vi "Read.vi"(8 "error in (no error)":errorcluster, 11 "Keithley 2100 in":refnum<class "Keithley 2100.lvclass">) -> (0 "error out":errorcluster, 1 "Unit":string, 2 "Measure":dbl, 3 "Keithley 2100 out":refnum<class "Keithley 2100.lvclass">, 4 "Channel":i32)   [LabVIEW 2020, in "Keithley 2100.lvclass"]
uses:
  Keithley 2100.lvclass
  C:/Sandbox/Git_Sandbox/WiSpry Test Framework source code (LV20)/WiSpry Test Framework/Instruments/Instrument.lvclass
  C:/Sandbox/Git_Sandbox/WiSpry Test Framework source code (LV20)/WiSpry Test Framework/Instruments/Digital Multimeter/Digital Multimeter.lvclass
  Digital Multimeter.lvclass/Digital Multimeter.ctl
  Instrument.lvclass/Instrument.ctl
  Instrument.lvclass
  <instrlib>/Keithley 2100 Series/Keithley 2100 Series.lvlib
  Digital Multimeter.lvclass
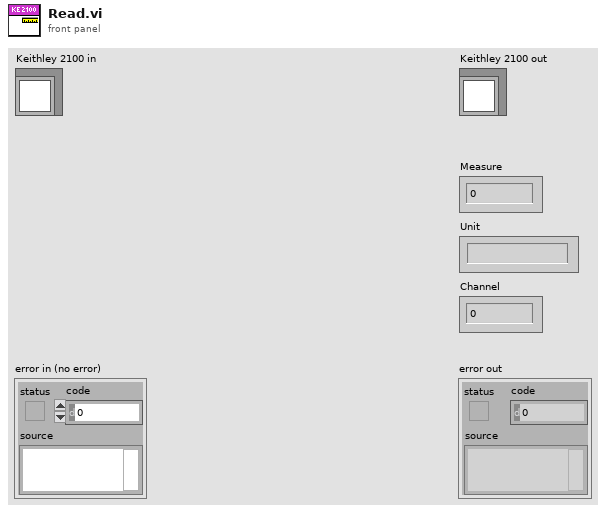
[diagram p1: front panel]
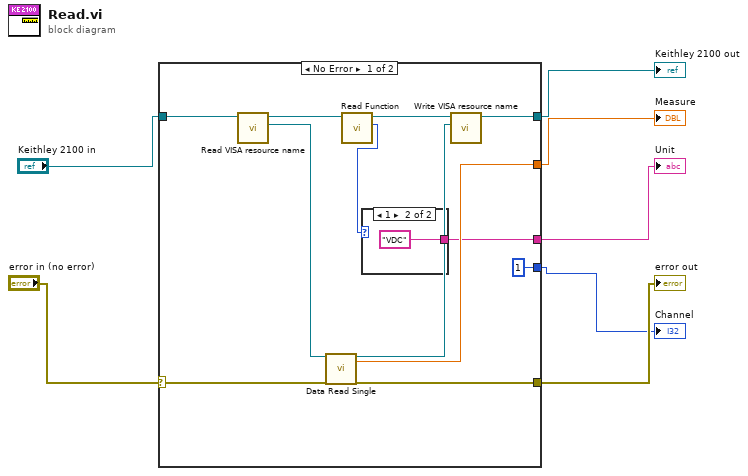
[diagram p0: block diagram]
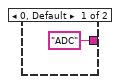
[diagram p2: hidden frame]
diagram:
  n1 = case shown="No Error" "error in (no error)" {
    selector: "error in (no error)" -> [w17 w23]
    tunnel: [w14 w23] -> w3
    tunnel: "Keithley 2100 in" -> [w19 w22]
    tunnel: [w18 w22] -> w4
    tunnel: [w13 _] -> w5
    tunnel: [1 ("Channel") _] -> w1
    tunnel: [w9 _] -> w2
    frame No Error {
      n2 = call "Read VISA resource name.vi"("Instrument in"=w19) -> ("VISA resource name"=w16:refnum<visa-resource-name>, "Instrument out"=w12:refnum<class "Keithley 2100.lvclass">)  [unwired: 9 in]
      n3 = call <instrlib>:"Data Read Single.vi"("VISA resource name"=w16, "error in (no error)"=w17) -> ("VISA resource name out"=w15:refnum<visa-resource-name>, "Measurement"=w13:dbl, "error out"=w14:errorcluster)  [unwired: 15 in]
      n4 = call "Read Function.vi"("Digtal Multimeter in"=w12) -> ("Function"=w10:u16, "Digtal Multimeter out"=w11:refnum<class "Keithley 2100.lvclass">)  [unwired: 9 in]
      n5 = case shown="1" w10 {
        tunnel: ["ADC" ("Unit") "VDC" ("Unit")] -> w9
        frame 0, Default {
        }
        frame 1 {
        }
      }
      n6 = call "Write VISA resource name.vi"("VISA resource name"=w15, "Instrument in"=w11) -> ("Instrument out"=w18:refnum<class "Keithley 2100.lvclass">)  [unwired: 9 in]
    }
    frame Error {
    }
  }
  "error out" <- w3
  "Keithley 2100 out" <- w4
  "Measure" <- w5
  "Unit" <- w2
  "Channel" <- w1
